vi "DDS9959 Set Clock.vi"(8 "error in (no error)":errorcluster, 9 "VCO Gain":bool, 10 "PLL Multiplier":u8, 11 "VISA resource name":refnum<visa-resource-name>) -> (0 "error out":errorcluster, 3 "VISA resource name out":refnum<visa-resource-name>)   [LabVIEW 2012]
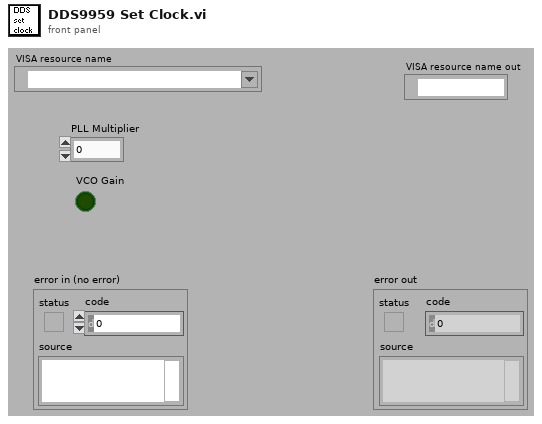
[diagram p1: front panel]
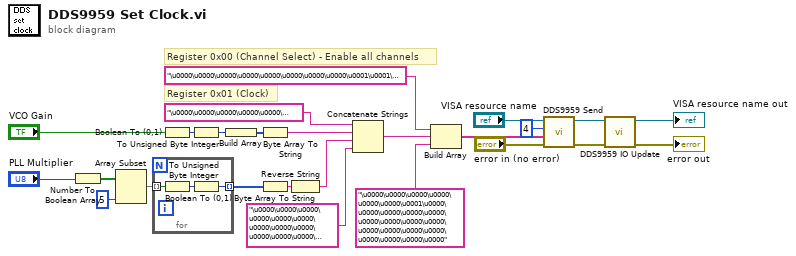
[diagram p0: block diagram]
diagram:
  # "Register 0x00 (Channel Select) - Enable all channels"
  # "Register 0x01 (Clock)"
  n1 = Number To Boolean Array(number="PLL Multiplier") -> (Boolean array=w17:bool[])
  n2 = Array Subset(array=w17, length=5) -> (w7:bool[])  [unwired: 1 in]
  n3 = for {
    tunnel: w7 -> [w28] mode=indexing
    tunnel: [w26] -> w9 mode=indexing
    n4 = Boolean To (0,1)(Boolean=w28) -> (0, 1=w27:i16)
    n5 = To Unsigned Byte Integer(number=w27) -> (unsigned 8bit integer=w26:u8)
  }
  n6 = Boolean To (0,1)(Boolean="VCO Gain") -> (0, 1=w14:i16)
  n7 = To Unsigned Byte Integer(number=w14) -> (unsigned 8bit integer=w12:u8)
  n8 = Build Array(w12) -> (w11:u8[])
  n9 = Byte Array To String(unsigned byte array=w11) -> (string=w10:string)
  n10 = Byte Array To String(unsigned byte array=w9) -> (string=w8:string)
  n11 = Reverse String(1:w8) -> (0:w6:string)
  n12 = Concatenate Strings("\u0000\u0000\u0000\u0000\u0000\u0000\u0000\u0001", w10, w6, "\u0000\u0000\u0000\u0000\u0000\u0000\u0000\u0000\u0000\u0000\u0000\u0000\u0000\u0000\u0000\u0000\u0000\u0000") -> (w20:string)
  n13 = Build Array("\u0000\u0000\u0000\u0000\u0000\u0000\u0000\u0000\u0001\u0001\u0001\u0001\u0000\u0000\u0000\u0000", w20, "\u0000\u0000\u0000\u0000\u0000\u0000\u0001\u0000\u0000\u0000\u0000\u0000\u0000\u0000\u0000\u0000\u0000\u0000\u0000\u0000\u0000\u0000\u0000\u0000") -> (w18:string[])
  n14 = call "DDS9959 Send.vi"("error in (no error)"="error in (no error)", "Output Array"=w18, "USB Out Endpoint"=i16 4, "VISA resource name"="VISA resource name") -> ("error out"=w3:errorcluster, "VISA resource name"=w4:refnum<visa-resource-name>)  [unwired: 6 in]
  n15 = call "DDS9959 IO Update.vi"("error in (no error)"=w3, "VISA resource name"=w4) -> ("error out"=→"error out":errorcluster, "VISA resource name out"=→"VISA resource name out":refnum<visa-resource-name>)  [unwired: 4 in]
